vi "Find Nearest Neighbors Index Byte.vi"(7 "#Neighbors":i32=1, 8 "error in (no error)":errorcluster, 10 "Points":u8[][](array[numeric]), 11 "KD Tree Byte in":refnum<class "KD Tree Byte.lvclass">) -> (0 "error out":errorcluster, 1 "Dists":sgl[][](array[numeric]), 2 "Indices":i32[][](array[numeric]), 3 "KD Tree Byte out":refnum<class "KD Tree Byte.lvclass">)   [LabVIEW 2020, in "KD Tree.lvlib" / "KD Tree Byte.lvclass"]
uses:
  KD Tree Byte.lvclass
  E:/Labview/LV 2020/Libs/flann/flann/Classes/KD Tree/KD Tree.lvclass
  KD Tree/KD Tree.lvclass/KD Tree.ctl
  KD Tree/Read index_ptr.vi
  KD Tree/Read flann_params.vi
  KD Tree/Read Overwrite Lib Path.vi
  KD Tree.lvlib
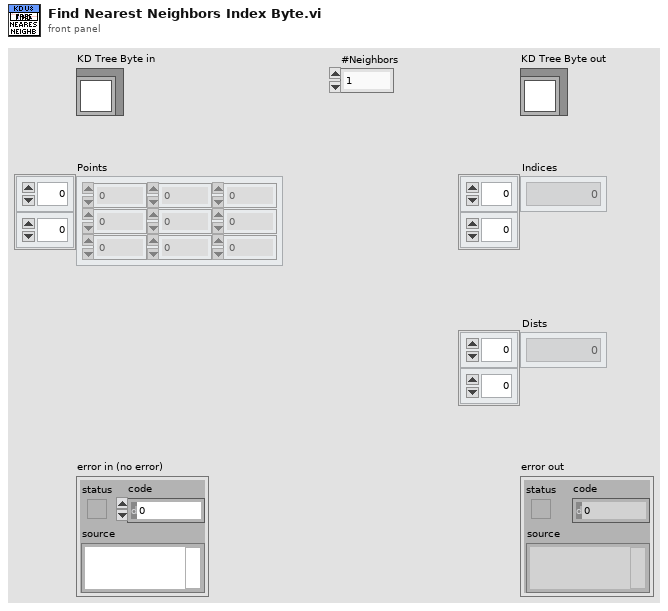
[diagram p1: front panel]
types:
  T1 = typedef "KD Tree.lvlib/Flann Params.ctl" = cluster{"algorithm":u32, "checks":i32, "eps":sgl, "sorted":i32, "max_neighbors":i32, "cores":i32, "trees":i32, "leaf_max_size":i32, "branching":i32, "iterations":i32, "centers_init":u32, "cb_index":sgl, "target_precision":sgl, "build_weight":sgl, "memory_weight":sgl, "sample_fraction":sgl, "table_number_":u32, "key_size_":u32, "multi_probe_level_":u32, "log_level":u32, "random_seed":i32}
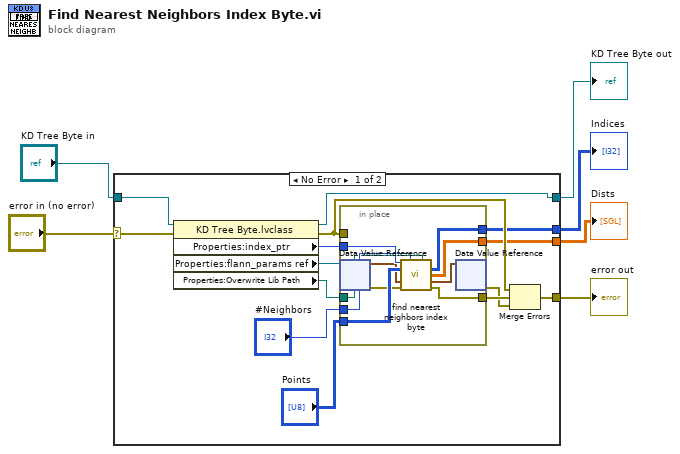
[diagram p0: block diagram]
diagram:
  n1 = case shown="No Error" "error in (no error)" {
    selector: "error in (no error)" -> [w20 w32]
    tunnel: [w13 w32] -> w5
    tunnel: [w18 w31] -> w3
    tunnel: "KD Tree Byte in" -> [w19 w31]
    tunnel: [w8 _] -> w2
    tunnel: [w7 _] -> w1
    frame No Error {
      n2 = property class="KD Tree Byte.lvclass"(reference=w19, error in=w20) -> (reference out=w18:refnum<class "KD Tree Byte.lvclass">, error out=w9:errorcluster, "Properties:index_ptr"=w17:u64, "Properties:flann_params ref"=w14:refnum<data-value>, "Properties:Overwrite Lib Path"=w10:path)
      n3 = in-place {
        in-place-border: w17 -> [w30]
        in-place-border: "#Neighbors" -> [w29]
        in-place-border: "Points" -> [w28]
        in-place-border: [w24] -> w8
        in-place-border: [w23] -> w7
        in-place-border: [w22] -> w12
        in-place-border: w10 -> [w21]
        in-place-border: w9 -> [_]
        n4 = in-place-dvr #1(w14) -> (w27:T1, w26:errorcluster)
        n5 = call "find nearest neighbors index byte.vi"("index_id"=w30, "nn"=w29, "Overwrite Lib Path"=w21, "testset"=w28, "flann_params"=w27, "error in (no error)"=w26) -> ("Indices"=w24:i32[][], "Dists"=w23:sgl[][], "flann_params"=w25:T1, "error out"=w22:errorcluster)  [unwired: 5 in, 1 out]
        n6 = in-place-dvr #1(w25) -> (w11:errorcluster)  [unwired: 1 out]
      }
      n7 = Merge Errors(w9, w12, w11) -> (w13:errorcluster)
    }
    frame Error {
    }
  }
  "error out" <- w5
  "KD Tree Byte out" <- w3
  "Indices" <- w2
  "Dists" <- w1
